vi "Version2.0.vi"() -> ()   [LabVIEW 2012]
uses:
  Function_Set/Debug/Function_Set.dll
panel:
  in  "Initial Folder Path:":path
  in  "选项卡控件":T1(tab)
  in  "Double:":dbl
  in  "String:":string
  in  "Other:":string
  in  "Save This Shot":bool
  out "Shots:":i32
  in  "Save This Notes":bool
  in  "Other Notes:":string
  in  "Options":u16(ring) caption="Choose File:" items=["2014-5-5-Notes.txt", "2014-5-5.txt"]
  in  "查询":bool
  out "Notes:":string
  out "Shots:":i32
  out "Shot's situation:":string
  in  "Your Own:":u16(ring) items=["2, 10000, 3, 1", "2, 10000, 4, 1"]
  in  "FrameStartTriggerMode":T2(ring)
  in  "AcquisitionMode":T3(ring)
  in  "ExposureMode":T4(ring)
  in  "AVT SDK Demon":bool
  out "CCD ID":string
  out "ExposureMode":string
  out "ExposureValue":u32
  out "AcquisitionMode":string
  out "FrameStartTriggerMode":string
  in  "ExposureValue":u32
  in  "CameraStart":bool
  in  "CameraStop":bool
  in  "CameraSet":bool
  in  "CameraGet":bool
  in  "CameraSetAll":bool
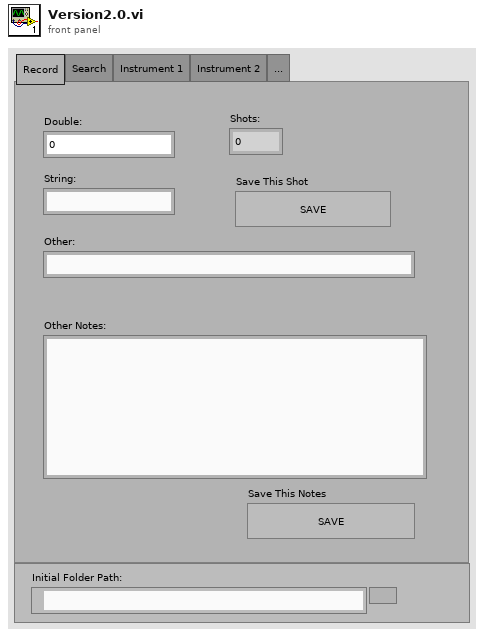
[diagram p1: front panel]
types:
  T1 = enum32{"Record", "Search", "Instrument 1", "Instrument 2", "..."}
  T2 = enum16{"默认", "Freerun", "SyncIn1", "SyncIn2", "FixedRate", "Software"}
  T3 = enum16{"默认", "Continuous", "SingleFrame", "MultiFrame", "Recorder"}
  T4 = enum16{"默认", "Manual", "Auto", "AutoOnce", "External"}
  T5 = enum16{"open", "replace", "create", "open or create", "replace or create", "replace or create with confirmation"}
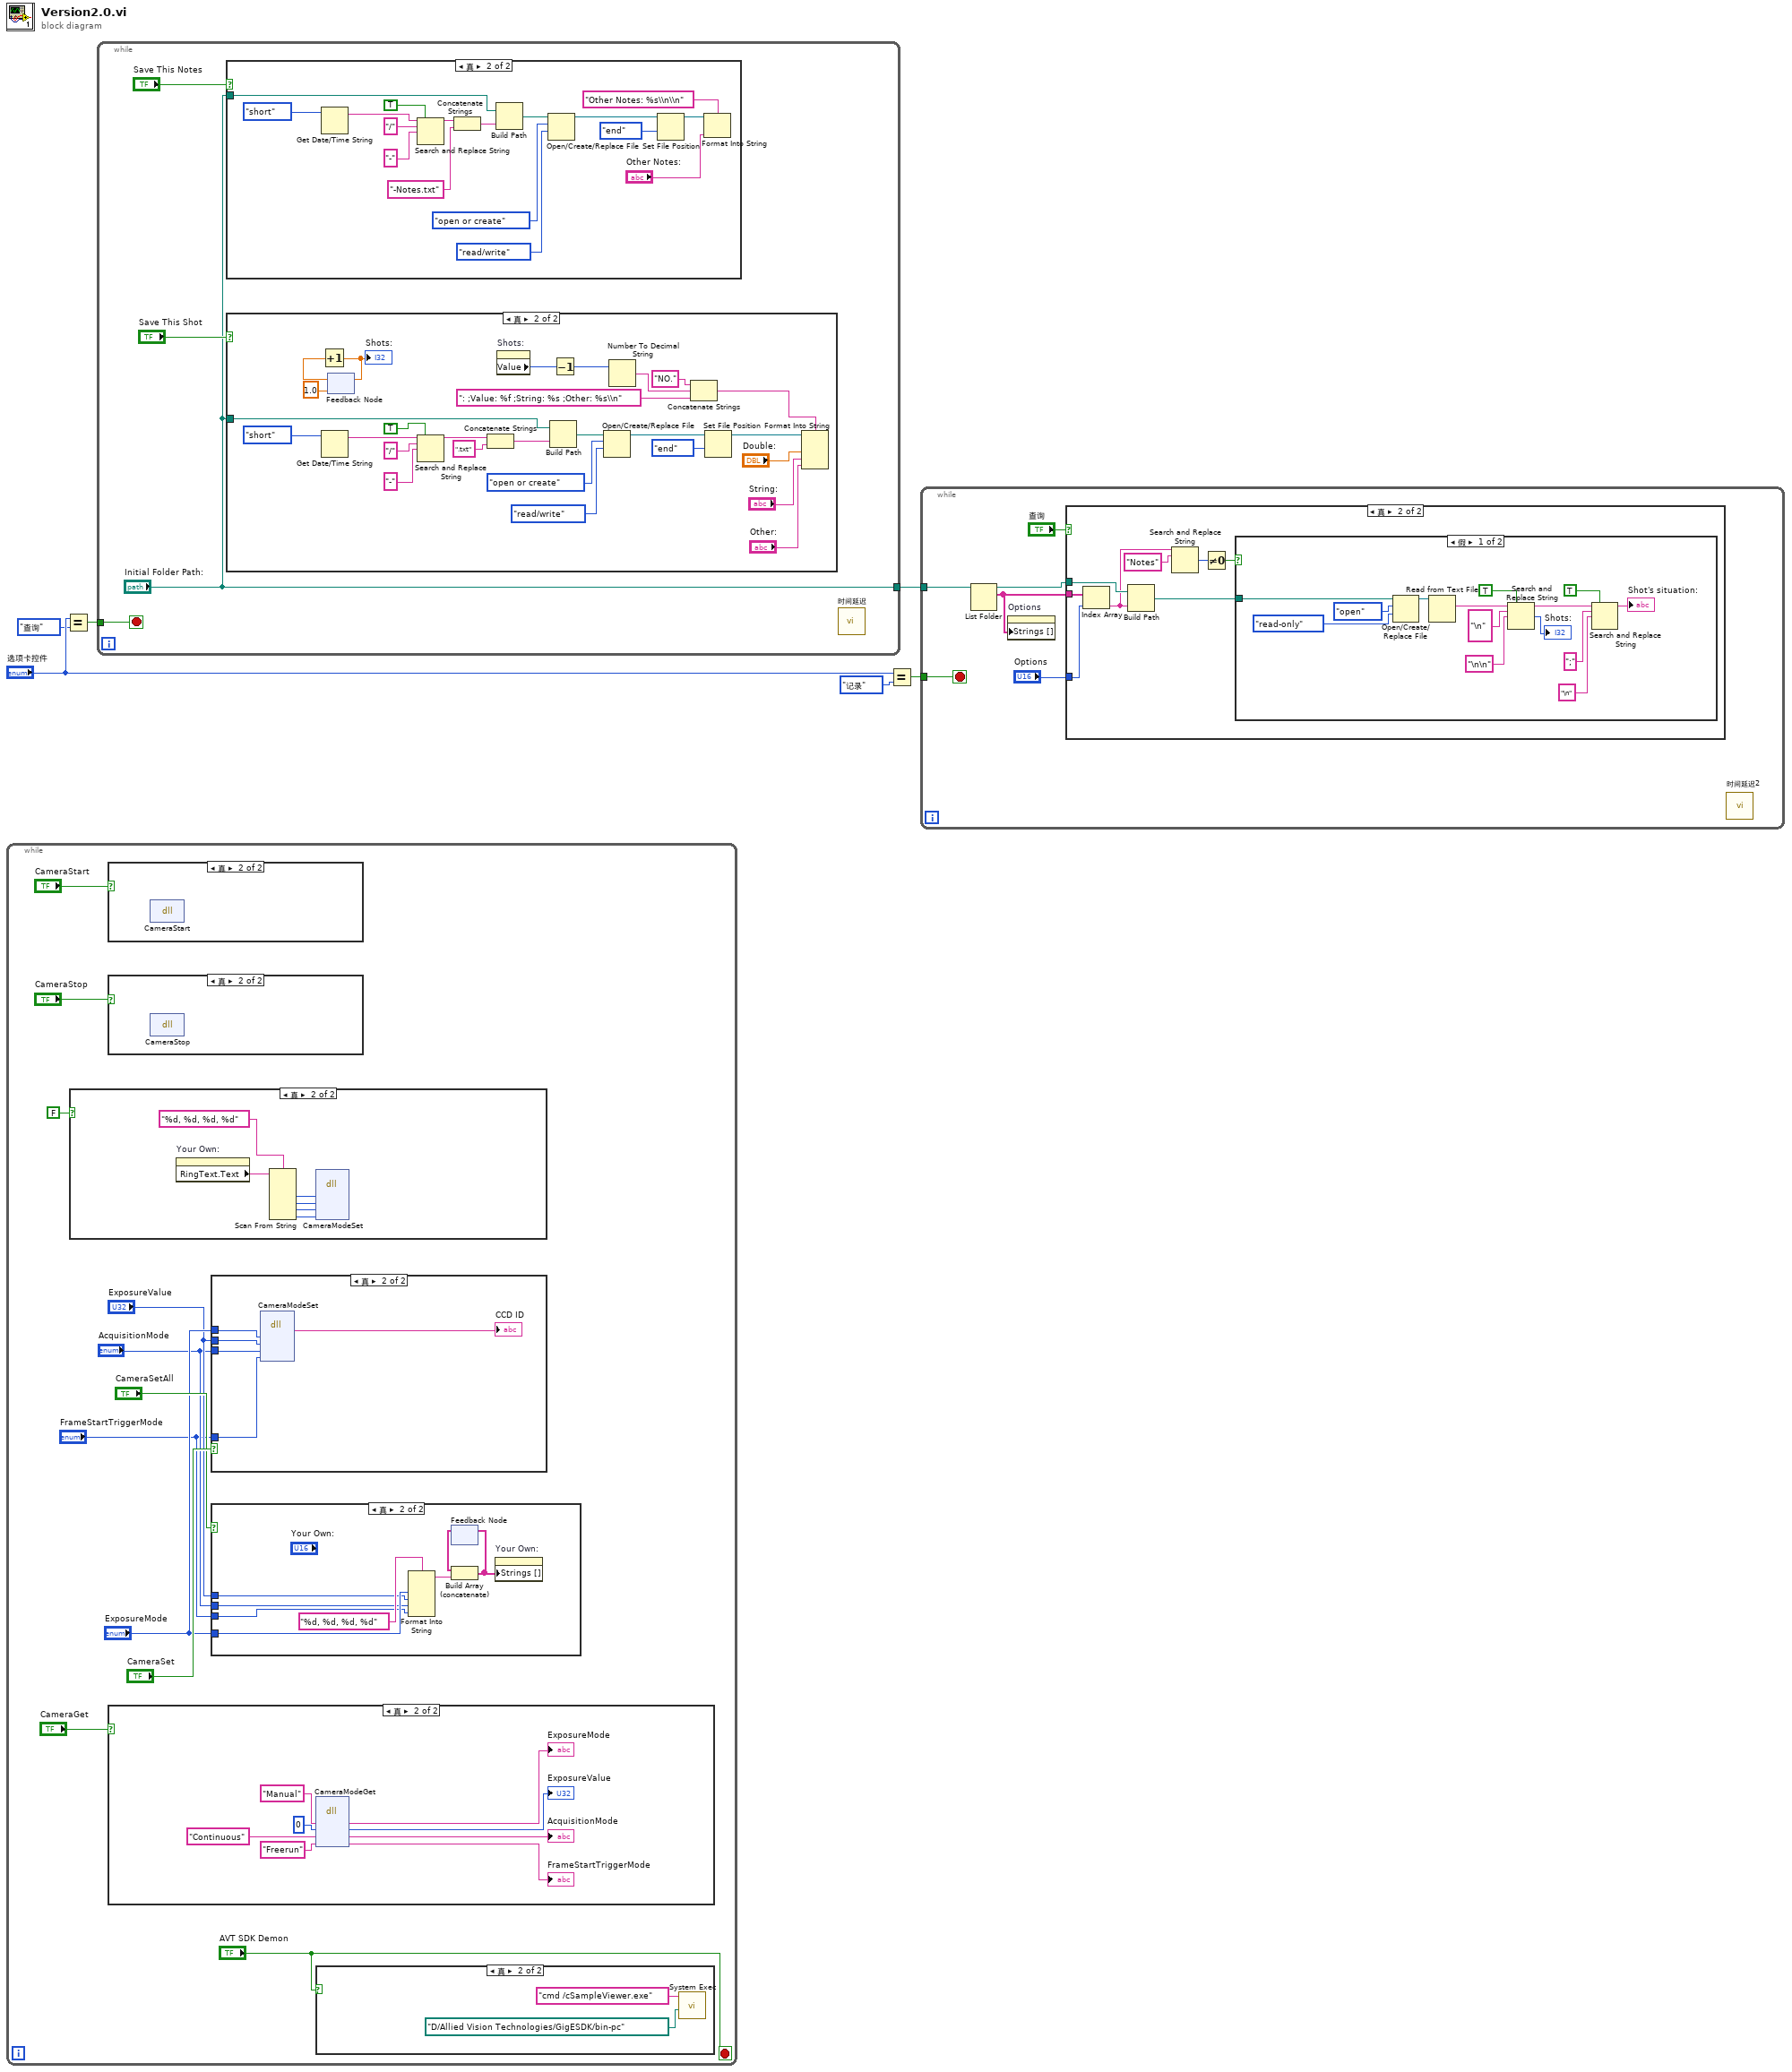
[diagram p0: block diagram]
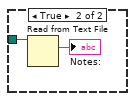
[diagram p10: hidden frame]
diagram:
  n1 = while {
    stop <- "AVT SDK Demon" stop-if-true
    n2 = case shown="真" FALSE {
      frame False {
      }
      frame True {
        n3 = property on="Your Own:" class="Ring (严格)"() -> ("RingText.Text"=w18:string)  [unwired: 2 in, 2 out]
        n4 = Scan From String(format string="%d, %d, %d, %d" ("格式字符串"), input string=w18) -> (output 1=w20:i32, output 2=w21:i32, output 3=w22:i32, output 4=w23:i32)  [unwired: 6 in, 3 out]
        n5 = dll-call lib="F:/Kun's Test/Function_Set/Debug/Function_Set.dll" fn="CameraModeSet"("EM"=w20, "EV"=w21, "AM"=w22, "FSTM"=w23) -> ()  [unwired: 8 in, 2 out]
      }
    }
    n6 = case shown="真" "CameraStart" {
      frame False {
      }
      frame True {
        n7 = dll-call lib="F:/Kun's Test/Function_Set/Debug/Function_Set.dll" fn="CameraStart"() -> ()  [unwired: 4 in, 2 out]
      }
    }
    n8 = case shown="真" "CameraStop" {
      frame False {
      }
      frame True {
        n9 = dll-call lib="F:/Kun's Test/Function_Set/Debug/Function_Set.dll" fn="CameraStop"() -> ()  [unwired: 4 in, 2 out]
      }
    }
    n10 = case shown="真" "CameraGet" {
      frame False {
      }
      frame True {
        n11 = dll-call lib="F:/Kun's Test/Function_Set/Debug/Function_Set.dll" fn="CameraModeGet"("ExposureMode"="Manual", "ExposureValue"=u32 0, "AcquisitionMode"="Continuous", "FrameStartTriggerMode"="Freerun") -> ("ExposureMode"=→"ExposureMode":string, "ExposureValue"=→"ExposureValue":u32, "AcquisitionMode"=→"AcquisitionMode":string, "FrameStartTriggerMode"=→"FrameStartTriggerMode":string)  [unwired: 4 in, 2 out]
      }
    }
    n12 = case shown="真" "CameraSet" {
      tunnel: "ExposureValue" -> [_ w43]
      tunnel: "ExposureMode" -> [_ w42]
      tunnel: "AcquisitionMode" -> [_ w41]
      tunnel: "FrameStartTriggerMode" -> [_ w40]
      frame False {
      }
      frame True {
        n13 = dll-call lib="F:/Kun's Test/Function_Set/Debug/Function_Set.dll" fn="CameraModeSet"("EM"=w42, "EV"=w43, "AM"=w41, "FSTM"=w40) -> ("返回类型"=→"CCD ID":string)  [unwired: 7 in, 2 out]
      }
    }
    n14 = case shown="真" "CameraSetAll" {
      tunnel: "ExposureMode" -> [_ w27]
      tunnel: "ExposureValue" -> [_ w26]
      tunnel: "AcquisitionMode" -> [_ w25]
      tunnel: "FrameStartTriggerMode" -> [_ w24]
      frame False {
      }
      frame True {
        n15 = Format Into String(format string="%d, %d, %d, %d" ("格式字符串"), w27, w26, w25, w24) -> (resulting string=w30:string)  [unwired: 2 in, 1 out]
        n16 = feedback #1() -> (w29:string[])  [unwired: 1 in]
        n17 = Build Array (concatenate)(w29, w30) -> (w28:string[])
        n18 = feedback-in #1(w28) -> ()
        n19 = property on="Your Own:" class="Ring (严格)"("Strings []"=w28) -> ()  [unwired: 2 in, 2 out]
      }
    }
    n20 = case shown="真" "AVT SDK Demon" {
      frame False {
      }
      frame True {
        n21 = call <vilib>:"System Exec.vi"("working directory"=path "D:/Allied Vision Technologies/GigESDK/bin-pc", "command line"="cmd /cSampleViewer.exe") -> ()  [unwired: 6 in, 4 out]
      }
    }
  }
  n22 = Equal?(x="选项卡控件", y=enum32{"记录", "查询"}."查询") -> (x = y?=w2:bool)
  n23 = while {
    tunnel: ["Initial Folder Path:"] -> w6
    tunnel: w2 -> [w47]
    stop <- w47 stop-if-true
    n24 = case shown="真" "Save This Notes" {
      tunnel: "Initial Folder Path:" -> [_ w51]
      frame False {
      }
      frame True {
        n25 = Get Date/Time String(date format (0)=enum16{"short", "long", "abbreviated"}."short" ("日期格式(0)")) -> (date string=w63:string)  [unwired: 2 in, 1 out]
        n26 = Search and Replace String(replace all?=TRUE ("替换全部？(F)"), input string=w63, search string="/" ("搜索字符串"), replace string="-" ("替换字符串(\"\")")) -> (result string=w54:string)  [unwired: 4 in, 3 out]
        n27 = Concatenate Strings(w54, "-Notes.txt" ("字符串")) -> (w52:string)
        n28 = Build Path(base path=w51, name or relative path=w52) -> (appended path=w64:path)
        n29 = Open/Create/Replace File(file path (use dialog)=w64, operation (0:open)=T5."open or create" ("操作(0:open)"), access (0:read/write)=enum16{"read/write", "read-only", "write-only"}."read/write" ("权限(0:read/write)")) -> (refnum out=w57:refnum<file>)  [unwired: 3 in, 2 out]
        n30 = Set File Position(refnum=w57, from (0:start)=enum16{"start", "end", "current"}."end" ("自（0:起始）")) -> (refnum out=w56:refnum<file>)  [unwired: 2 in, 1 out]
        n31 = Format Into String(format string="Other Notes: %s\\n\\n" ("格式字符串"), initial string=w56, "Other Notes:") -> ()  [unwired: 1 in, 2 out]
      }
    }
    n32 = case shown="真" "Save This Shot" {
      tunnel: "Initial Folder Path:" -> [_ w74]
      frame False {
      }
      frame True {
        n33 = Get Date/Time String(date format (0)=enum16{"short", "long", "abbreviated"}."short" ("日期格式(0)")) -> (date string=w88:string)  [unwired: 2 in, 1 out]
        n34 = feedback #2(1.0 ("x")) -> (w77:dbl)
        n35 = Increment(x=w77) -> (x+1=w75:dbl)
        "Shots:" <- w75
        n36 = feedback-in #2(w75) -> ()
        n37 = Search and Replace String(replace all?=TRUE ("替换全部？(F)"), input string=w88, search string="/" ("搜索字符串"), replace string="-" ("替换字符串(\"\")")) -> (result string=w85:string)  [unwired: 4 in, 3 out]
        n38 = Concatenate Strings(w85, ".txt" ("字符串")) -> (w90:string)
        n39 = property on="Shots:" class="DigNum (严格)"() -> ("Value"=w69:i32)  [unwired: 2 in, 2 out]
        n40 = Build Path(base path=w74, name or relative path=w90) -> (appended path=w91:path)
        n41 = Decrement(x=w69) -> (x-1=w68:i32)
        n42 = Open/Create/Replace File(file path (use dialog)=w91, operation (0:open)=T5."open or create" ("操作(0:open)"), access (0:read/write)=enum16{"read/write", "read-only", "write-only"}."read/write" ("权限(0:read/write)")) -> (refnum out=w79:refnum<file>)  [unwired: 3 in, 2 out]
        n43 = Number To Decimal String(number=w68) -> (decimal integer string=w73:string)  [unwired: 1 in]
        n44 = Concatenate Strings("NO." ("字符串"), w73, ": ;Value: %f ;String: %s ;Other: %s\\n" ("格式字符串")) -> (w70:string)
        n45 = Set File Position(refnum=w79, from (0:start)=enum16{"start", "end", "current"}."end" ("自（0:起始）")) -> (refnum out=w78:refnum<file>)  [unwired: 2 in, 1 out]
        n46 = Format Into String(format string=w70, initial string=w78, "Double:", "String:", "Other:") -> ()  [unwired: 1 in, 2 out]
      }
    }
    n47 = call "时间延迟"() -> ()  [unwired: 11 in, 1 out]
  }
  n48 = Equal?(x="选项卡控件", y=enum32{"记录", "查询"}."记录") -> (x = y?=w1:bool)
  n49 = while {
    tunnel: w6 -> [w100]
    tunnel: w1 -> [w95]
    stop <- w95 stop-if-true
    n50 = List Folder(path=w100) -> (path out=w97:path, filenames=w99:string[])  [unwired: 3 in, 2 out]
    n51 = property on="Options" class="Ring (严格)"("Strings []"=w99) -> ()  [unwired: 2 in, 2 out]
    n52 = case shown="真" "查询" {
      tunnel: w99 -> [_ w108]
      tunnel: "Options" -> [_ w107]
      tunnel: w97 -> [_ w106]
      frame False {
      }
      frame True {
        n53 = Index Array(array=w108, index=w107) -> (element=w105:string)
        n54 = Build Path(base path=w106, name or relative path=w105) -> (appended path=w101:path)
        n55 = Search and Replace String(input string=w105, search string="Notes" ("搜索字符串")) -> (number of replacements=w103:i32)  [unwired: 6 in, 3 out]
        n56 = Not Equal To 0?(x=w103) -> (x != 0?=w102:bool)
        n57 = case shown="假" w102 {
          tunnel: w101 -> [w122 w124]
          frame False {
            n58 = Open/Create/Replace File(file path (use dialog)=w122, operation (0:open)=T5."open" ("操作(0:open)"), access (0:read/write)=enum16{"read/write", "read-only", "write-only"}."read-only" ("权限(0:read/write)")) -> (refnum out=w119:refnum<file>)  [unwired: 3 in, 2 out]
            n59 = Read from Text File(file (use dialog)=w119) -> (text=w115:string)  [unwired: 3 in, 3 out]
            n60 = Search and Replace String(replace all?=TRUE ("替换全部？(F)"), input string=w115, search string="\n" ("搜索字符串"), replace string="\n\n" ("替换字符串(\"\")")) -> (result string=w112:string, number of replacements=→"Shots:":i32)  [unwired: 4 in, 2 out]
            n61 = Search and Replace String(replace all?=TRUE ("替换全部？(F)"), input string=w112, search string=";" ("搜索字符串"), replace string="\n" ("替换字符串(\"\")")) -> (result string=→"Shot's situation:":string)  [unwired: 4 in, 3 out]
          }
          frame True {
            n62 = Read from Text File(file (use dialog)=w124) -> (text=→"Notes:":string)  [unwired: 3 in, 3 out]
          }
        }
      }
    }
    n63 = call "时间延迟2"() -> ()  [unwired: 11 in, 1 out]
  }
